vi "RxPkt - Init Packet Page.vi"(7 "Rx Section Cluster In":T2, 8 "error in (no error)":errorcluster, 11 "Node Ptr In":T1 format="%.0x") -> (0 "error out":errorcluster, 3 "Node Ptr Out":T1 format="%.0x", 5 "Rx Section Cluster Out":T2)   [LabVIEW 2023, in "UDP-Custom-Device System Explorer.lvlib"]
uses:
  UDP-Custom-Device System Explorer.lvlib
  Types/Page References/Refs - Rx Packets Page.ctl
  <vilib>/NI VeriStand/Custom Device API/Custom Device Item Ref.ctl
  <vilib>/NI VeriStand/Custom Device API/Custom Device API.lvlib
  Property Accessors/Shared Packet Accessors.lvlib
  Property Accessors/Rx Channel Section Accessors.lvlib
  Property Accessors/Rx Packet Accessors.lvlib
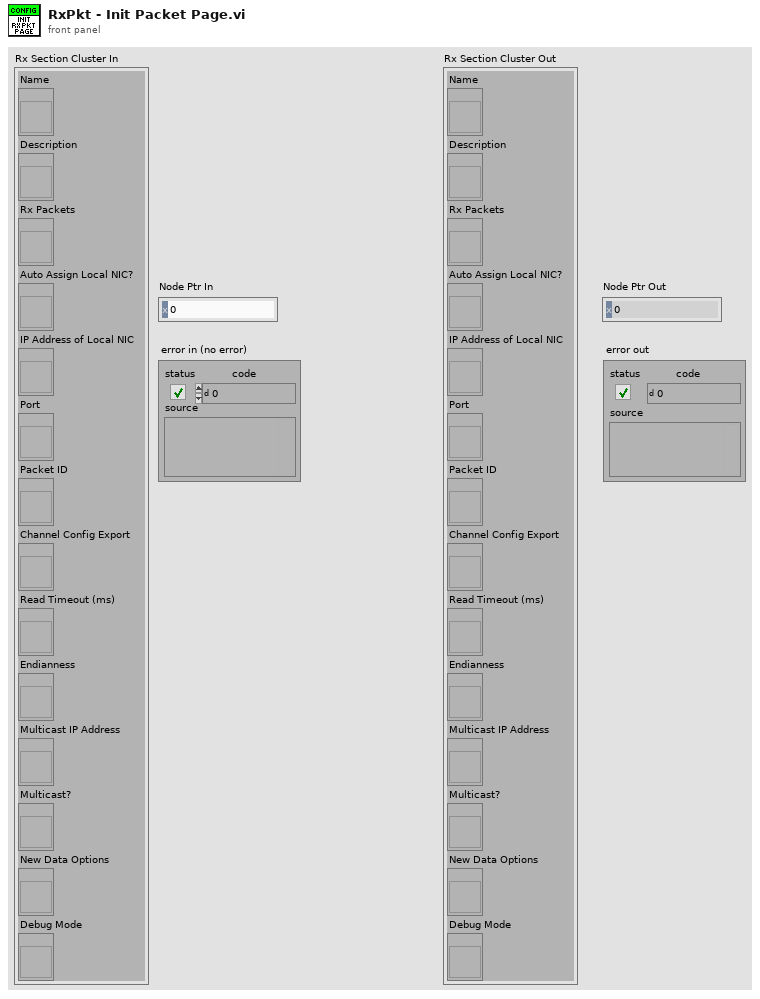
[diagram p1: front panel]
types:
  T1 = typedef "Custom Device API.lvlib/Custom Device Item Ref.ctl" = u64
  T2 = typedef "UDP-Custom-Device System Explorer.lvlib/Refs - Rx Packets Page.ctl" = cluster{"Name":refnum<vi>, "Description":refnum<vi>, "Rx Packets":refnum<vi>, "Auto Assign Local NIC?":refnum<vi>, "IP Address of Local NIC":refnum<vi>, "Port":refnum<vi>, "Packet ID":refnum<vi>, "Channel Config Export":refnum<vi>, "Read Timeout (ms)":refnum<vi>, "Endianness":refnum<vi>, "Multicast IP Address":refnum<vi>, "Multicast?":refnum<vi>, "New Data Options":refnum<vi>, "Debug Mode":refnum<vi>}
  T3 = enum8{"Enabled", "Disabled", "Disabled and Grayed Out"}
  T4 = typedef "UDP-Custom-Device Shared.lvlib/Shared - New Data Options.ctl" = enum16{"Timeout Reset", "Counter"}
  T5 = typedef "Custom Device API.lvlib/Custom Device Item Info.ctl" = cluster{"Name":string, "Is Channel":bool, "GUID":string, "Is Waveform":bool}
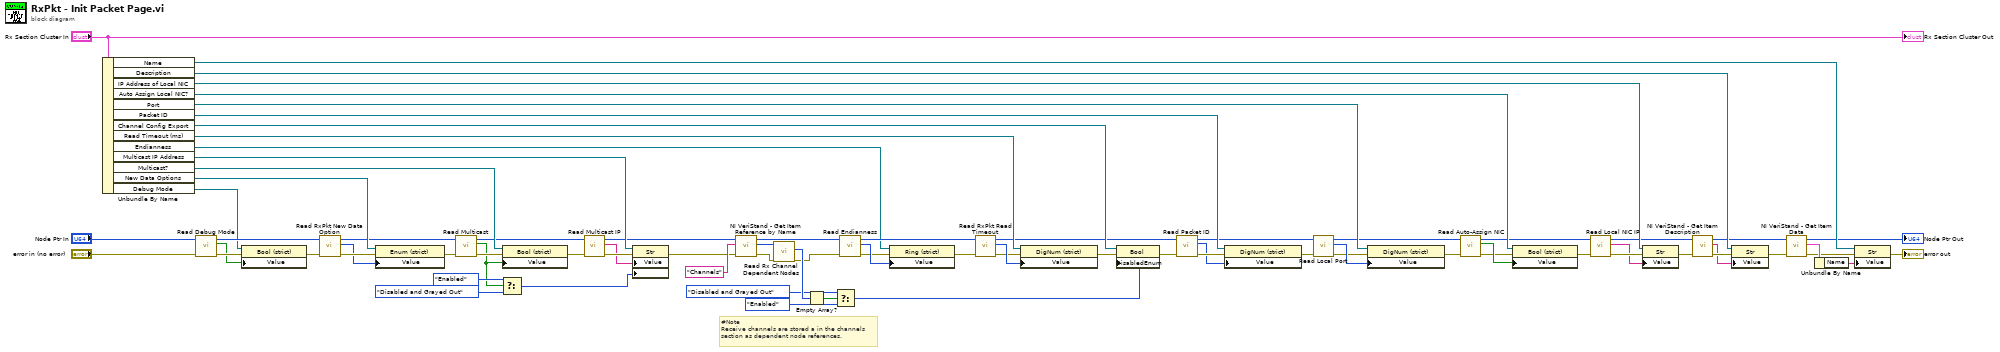
[diagram p0: block diagram]
diagram:
  # "#Note\nReceive channels are stored a in the channels\nsection as dependent node references."
  n1 = Unbundle By Name("Rx Section Cluster In") -> ("Name"=w75:refnum<vi>, "Description"=w74:refnum<vi>, "IP Address of Local NIC"=w64:refnum<vi>, "Auto Assign Local NIC?"=w65:refnum<vi>, "Port"=w76:refnum<vi>, "Packet ID"=w77:refnum<vi>, "Channel Config Export"=w47:refnum<vi>, "Read Timeout (ms)"=w37:refnum<vi>, "Endianness"=w29:refnum<vi>, "Multicast IP Address"=w23:refnum<vi>, "Multicast?"=w25:refnum<vi>, "New Data Options"=w12:refnum<vi>, "Debug Mode"=w1:refnum<vi>)
  n2 = call "Read Debug Mode.vi"("error in (no error)"="error in (no error)", "Node Ptr"="Node Ptr In") -> ("error out"=w7:errorcluster, "Debug Mode"=w6:bool, "Node Ptr out"=w4:T1)  [unwired: 7 in]
  n3 = property class="Bool (strict)"(reference=w1, error in=w7, "Value"=w6) -> (error out=w2:errorcluster)  [unwired: 1 out]
  n4 = call "Read RxPkt New Data Option.vi"("error in (no error)"=w2, "Node Ptr"=w4) -> ("error out"=w9:errorcluster, "New Data Option"=w8:T4, "Node Ptr out"=w10:T1)  [unwired: 7 in]
  n5 = property class="Enum (strict)"(reference=w12, error in=w9, "Value"=w8) -> (error out=w11:errorcluster)  [unwired: 1 out]
  n6 = call "Read Multicast.vi"("error in (no error)"=w11, "Node Ptr"=w10) -> ("error out"=w24:errorcluster, "Multicast"=w13:bool, "Node Ptr out"=w21:T1)  [unwired: 7 in]
  n7 = Select(t=T3."Enabled" ("Disabled"), s=w13, f=T3."Disabled and Grayed Out" ("Disabled")) -> (s? t:f=w14:T3)
  n8 = property class="Bool (strict)"(reference=w25, error in=w24, "Value"=w13) -> (error out=w19:errorcluster)  [unwired: 1 out]
  n9 = call "Read Multicast IP.vi"("error in (no error)"=w19, "Node Ptr"=w21) -> ("error out"=w18:errorcluster, "Multicast IP Address"=w17:string, "Node Ptr out"=w20:T1)  [unwired: 7 in]
  n10 = property class="Str"(reference=w23, error in=w18, "Value"=w17, "DisabledEnum"=w14) -> (error out=w22:errorcluster)  [unwired: 1 out]
  n11 = call <vilib>:"NI VeriStand - Get Item Reference by Name.vi"("error in (no error)"=w22, "Item Name"="Channels" ("Section Name"), "Parent Ref in"=w20) -> ("error out"=w43:errorcluster, "Item Ref"=w44:T1, "Parent Ref out"=w32:T1)  [unwired: 5 in, 1 out]
  n12 = call "Read Rx Channel Dependent Nodes.vi"("error in (no error)"=w43, "Node Ptr"=w44) -> ("error out"=w30:errorcluster, "Dependent Node Refs"=w42:T1[])  [unwired: 7 in, 1 out]
  n13 = Empty Array?(array=w42) -> (empty?=w39:bool)
  n14 = Select(t=T3."Disabled and Grayed Out" ("Disabled"), s=w39, f=T3."Enabled" ("Disabled")) -> (s? t:f=w38:T3)
  n15 = call "Read Endianness.vi"("error in (no error)"=w30, "Node Ptr"=w32) -> ("error out"=w27:errorcluster, "Endianness"=w28:u16, "Node Ptr out"=w31:T1)  [unwired: 7 in]
  n16 = property class="Ring (strict)"(reference=w29, error in=w27, "Value"=w28) -> (error out=w26:errorcluster)  [unwired: 1 out]
  n17 = call "Read RxPkt Read Timeout.vi"("error in (no error)"=w26, "Node Ptr"=w31) -> ("error out"=w34:errorcluster, "Read Timeout"=w36:i32, "Node Ptr out"=w35:T1)  [unwired: 7 in]
  n18 = property class="DigNum (strict)"(reference=w37, error in=w34, "Value"=w36) -> (error out=w33:errorcluster)  [unwired: 1 out]
  n19 = property class="Bool"(reference=w47, error in=w33, "DisabledEnum"=w38) -> (error out=w46:errorcluster)  [unwired: 1 out]
  n20 = call "Read Packet ID.vi"("error in (no error)"=w46, "Node Ptr"=w35) -> ("error out"=w62:errorcluster, "Packet ID"=w61:i32, "Node Ptr out"=w60:T1)  [unwired: 7 in]
  n21 = property class="DigNum (strict)"(reference=w77, error in=w62, "Value"=w61) -> (error out=w59:errorcluster)  [unwired: 1 out]
  n22 = call "Read Local Port.vi"("error in (no error)"=w59, "Node Ptr"=w60) -> ("error out"=w57:errorcluster, "Port"=w58:u16, "Node Ptr out"=w56:T1)  [unwired: 7 in]
  n23 = property class="DigNum (strict)"(reference=w76, error in=w57, "Value"=w58) -> (error out=w54:errorcluster)  [unwired: 1 out]
  n24 = call "Read Auto-Assign NIC.vi"("error in (no error)"=w54, "Node Ptr"=w56) -> ("error out"=w53:errorcluster, "Auto-Assign NIC"=w55:bool, "Node Ptr out"=w52:T1)  [unwired: 7 in]
  n25 = property class="Bool (strict)"(reference=w65, error in=w53, "Value"=w55) -> (error out=w51:errorcluster)  [unwired: 1 out]
  n26 = call "Read Local NIC IP.vi"("error in (no error)"=w51, "Node Ptr"=w52) -> ("error out"=w50:errorcluster, "IP Address of Local NIC"=w48:string, "Node Ptr out"=w49:T1)  [unwired: 7 in]
  n27 = property class="Str"(reference=w64, error in=w50, "Value"=w48) -> (error out=w63:errorcluster)  [unwired: 1 out]
  n28 = call <vilib>:"NI VeriStand - Get Item Description.vi"("error in (no error)"=w63, "Item Ref in"=w49) -> ("error out"=w73:errorcluster, "Description"=w72:string, "Item Ref out"=w70:T1)  [unwired: 7 out]
  n29 = property class="Str"(reference=w74, error in=w73, "Value"=w72) -> (error out=w71:errorcluster)  [unwired: 1 out]
  n30 = call <vilib>:"NI VeriStand - Get Item Data.vi"("error in (no error)"=w71, "Item Ref in"=w70) -> ("error out"=w78:errorcluster, "Item Info"=w79:T5, "Item Ref out"=→"Node Ptr Out":T1)  [unwired: 6 in, 1 out]
  n31 = Unbundle By Name(w79) -> ("Name"=w69:string)
  n32 = property class="Str"(reference=w75, error in=w78, "Value"=w69) -> (error out=→"error out":errorcluster)  [unwired: 1 out]
  "Rx Section Cluster Out" <- "Rx Section Cluster In"
